vi "Read Encoder Number Samples to Average.vi"(8 "error in (no error)":errorcluster, 11 "DriveMotors in":refnum<class "DriveMotors.lvclass">) -> (0 "error out":errorcluster, 2 "Encoder Number Samples to Average":u8=2 min=1 max=128, 3 "DriveMotors out":refnum<class "DriveMotors.lvclass">)   [LabVIEW 2013, in "DriveMotors.lvclass"]
uses:
  DriveMotors.lvclass
  DriveMotors.lvclass/DriveMotors.ctl
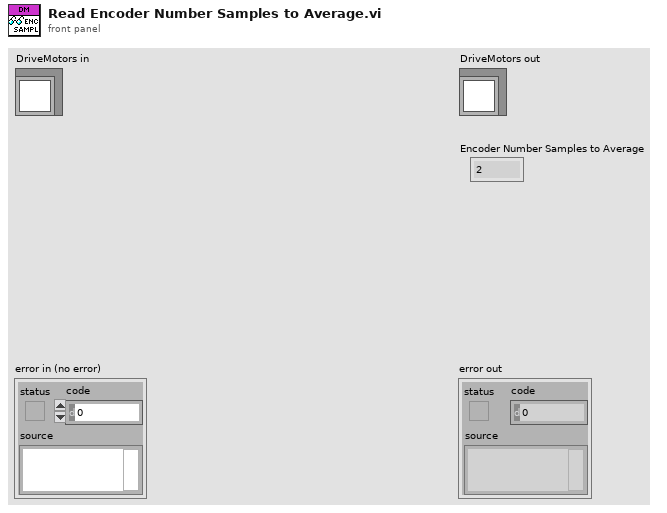
[diagram p1: front panel]
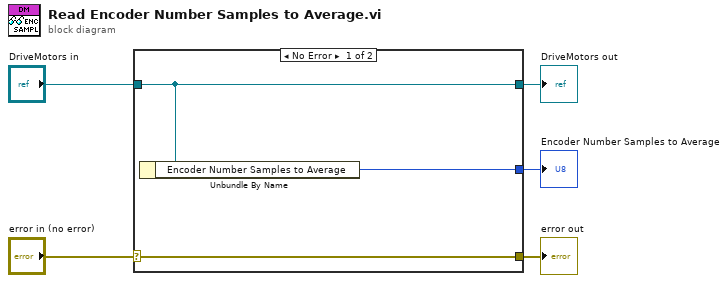
[diagram p0: block diagram]
diagram:
  n1 = case shown="No Error" "error in (no error)" {
    selector: "error in (no error)" -> [w8 w9]
    tunnel: [w8 w9] -> w4
    tunnel: [w7 w10] -> w2
    tunnel: "DriveMotors in" -> [w7 w10]
    tunnel: [w6 _] -> w1
    frame No Error {
      n2 = Unbundle By Name(w7) -> ("Encoder Number Samples to Average"=w6:u8)
    }
    frame Error {
    }
  }
  "error out" <- w4
  "DriveMotors out" <- w2
  "Encoder Number Samples to Average" <- w1
